vi "Render Missing Variable Key in Section.vi"(8 "Error In":errorcluster) -> (0 "Error Out":errorcluster)   [LabVIEW 2018, in "Tests.lvlib" / "Render.lvlib"]
uses:
  Render.lvlib
  <vilib>/addons/_JKI Toolkits/Caraya/classes/Test/Test.lvclass
  <vilib>/addons/_JKI Toolkits/Caraya/classes/Assert/Assert.lvclass
  src/Toolkit/Data/Map/Map.lvclass
  src/Toolkit/Low-Level/Support/Lex String.vi
  src/Toolkit/Data/Pair/Pair.lvclass
  src/Toolkit/Data/Pair/Support/From String.vi
  src/Toolkit/Data/Map/Support/From Pair Array.vi
  src/Toolkit/Low-Level/Renderer/Abstract/Render to String.vi
  src/Toolkit/Data/Boolean/Boolean.lvclass
  src/Toolkit/Data/Pair/Support/From Datum.vi
  src/Toolkit/Low-Level/Compiler/Compiler.lvclass
  D:/Users/cfield/Code/Field R&D Services/Labstache/src/Toolkit/Data/Datum/Datum.lvclass
  src/Toolkit/Low-Level/Nodes/Root/Root.lvclass
  D:/Users/cfield/Code/Field R&D Services/Labstache/src/Toolkit/Low-Level/Nodes/NonTerminal/NonTerminal.lvclass
  D:/Users/cfield/Code/Field R&D Services/Labstache/src/Toolkit/Low-Level/Nodes/Node/Node.lvclass
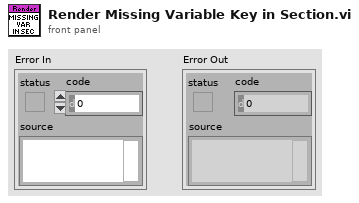
[diagram p1: front panel]
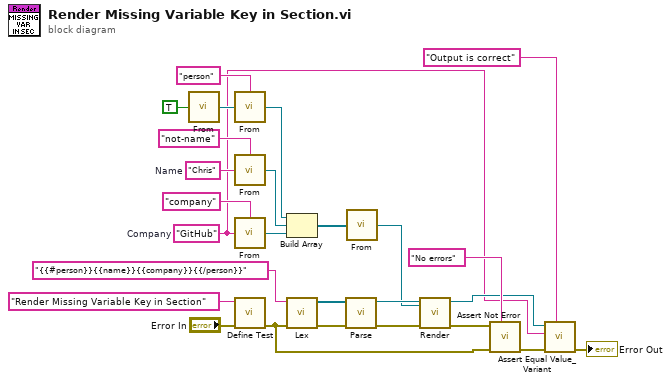
[diagram p0: block diagram]
diagram:
  w1 = "GitHub"  # Company
  w11 = "Chris"  # Name
  n1 = call "From.vi"("Value"=TRUE) -> ("Boolean"=w5:refnum<class "Boolean.lvclass">)
  n2 = call-poly "From.vi"("Value"=w5, "Key"="person") -> ("Pair"=w3:refnum<class "Pair.lvclass">)
  n3 = call-poly "From.vi"("Value"=w11, "Key"="not-name") -> ("Pair"=w9:refnum<class "Pair.lvclass">)
  n4 = call-poly "From.vi"("Value"=w1, "Key"="company") -> ("Pair"=w8:refnum<class "Pair.lvclass">)
  n5 = call <vilib>:"Define Test.vi"("error in (no error)"="Error In", "Label (VI Title)"="Render Missing Variable Key in Section") -> ("error out"=w13:errorcluster)  [unwired: 9 in]
  n6 = Build Array(w3, w9, w8) -> (w7:refnum<class "Pair.lvclass">[])
  n7 = call-poly "Lex.vi"("Error In"=w13, "Input"="{{#person}}{{name}}{{company}}{{/person}}" ("format string")) -> ("Error Out"=w16:errorcluster, "Tokens"=w17:refnum<class "Token.lvclass">[])  [unwired: 8 in]
  n8 = call "Parse.vi"("Error In"=w16, "Tokens"=w17) -> ("Error Out"=w18:errorcluster, "Abstract Syntax Tree"=w15:refnum<class "Root.lvclass">)  [unwired: 8 in]
  n9 = call-poly "From.vi"("Pairs"=w7) -> ("Map"=w2:refnum<class "Map.lvclass">)  [unwired: 1 in]
  n10 = call-poly "Render.vi"(7:w2, "Error In"=w18, "Context In"=w15) -> ("Error Out"=w20:errorcluster, "Context Out"=w19:refnum<class "Compiler.lvclass">)  [unwired: 6 in, 1 out]
  n11 = call <vilib>:"Assert Not Error.vi"("Label"="No errors", "error in (no error)"=w13, "Not Error?"=w20) -> ("error out"=w23:errorcluster)  [unwired: 8 in]
  n12 = call <vilib>:"Assert Equal Value_Variant.vi"("Label"="Output is correct", "error in (no error)"=w23, "Y"=w1, "X"=w19) -> ("error out"=→"Error Out":errorcluster)  [unwired: 7 in]
